vi "Read Data.vi"(8 "error in (no error)":errorcluster, 9 "Timeout in ms (-1)":i32=-1, 11 "Network Interface":refnum<data-value>) -> (0 "error out":errorcluster, 1 "Timed Out?":bool, 2 "Read Data":string, 3 "Network Interface Out":refnum<data-value>)   [LabVIEW 2019, in "Network Interface.lvlib" / "Network Interface.lvclass"]
uses:
  <vilib>/gpm_packages/@cs/Network-Sink/Source/Network Interface/Network Interface/Network Interface.lvclass
  <vilib>/gpm_packages/@cs/Network-Sink/Source/Network Interface/Network Interface/Network Interface.lvclass/Network Interface.ctl
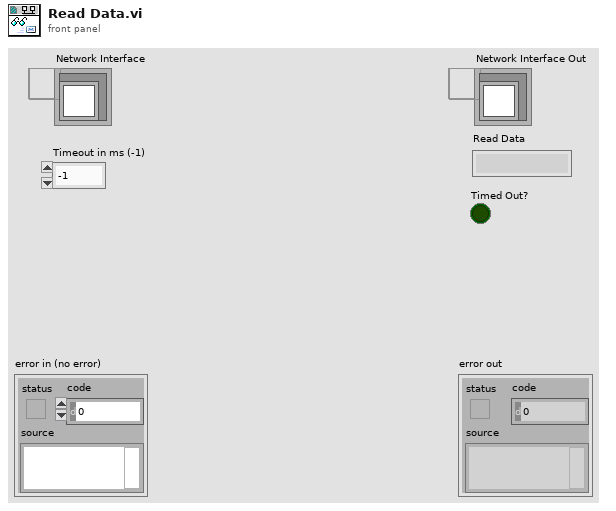
[diagram p1: front panel]
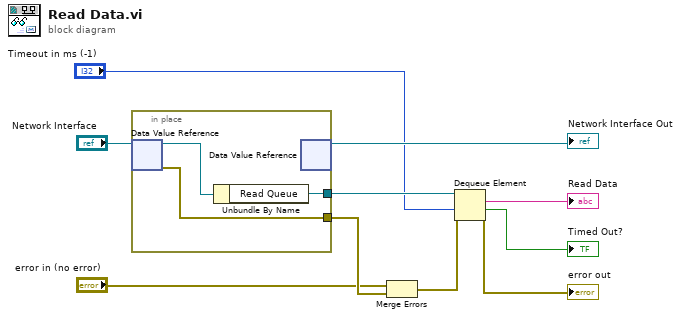
[diagram p0: block diagram]
diagram:
  n1 = in-place {
    in-place-border: [w12] -> w8
    in-place-border: [w11] -> w7
    n2 = in-place-dvr #1("Network Interface") -> (w13:refnum<class "Network Interface.lvclass">, w11:errorcluster)
    n3 = Unbundle By Name(w13) -> ("Read Queue"=w12:refnum<queue>)
    n4 = in-place-dvr #1() -> (→"Network Interface Out":refnum<data-value>)  [unwired: 1 in, 1 out]
  }
  n5 = Merge Errors("error in (no error)", w7) -> (w6:errorcluster)
  n6 = Dequeue Element(queue=w8, timeout in ms (-1)="Timeout in ms (-1)", error in (no error)=w6) -> (element=→"Read Data":string, timed out?=→"Timed Out?":bool, error out=→"error out":errorcluster)  [unwired: 1 out]
